vi "Log.vi"(8 "error in (no error)":errorcluster, 10 "Log Text":string, 11 "TDMS in":refnum<class "TDMS Sink.lvclass">) -> (0 "error out":errorcluster, 3 "TDMS out":refnum<class "TDMS Sink.lvclass">)   [LabVIEW 2020, in "LV Log.lvlib" / "TDMS Sink.lvclass"]
uses:
  TDMS Sink.lvclass
  TDMS Sink.lvclass/TDMS Sink.ctl
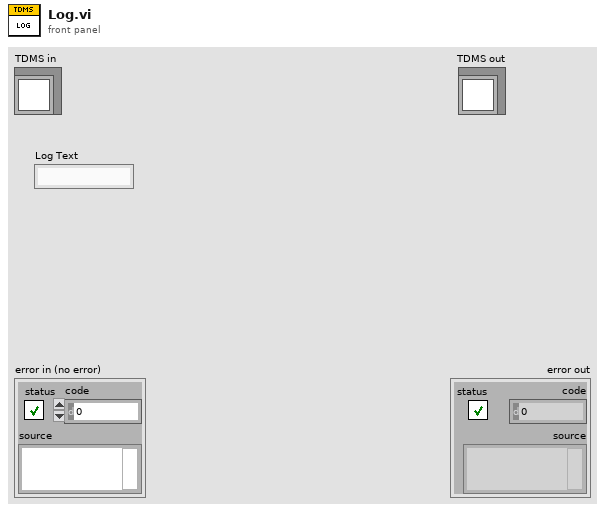
[diagram p1: front panel]
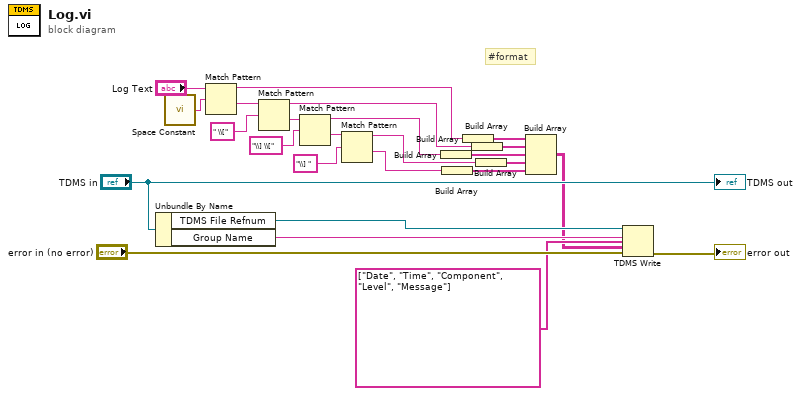
[diagram p0: block diagram]
diagram:
  # "#format"
  n1 = Unbundle By Name("TDMS in") -> ("TDMS File Refnum"=w22:refnum<k34>, "Group Name"=w21:string)
  n2 = call <vilib>:"Space Constant.vi"() -> ("String"=w12:string)
  n3 = Match Pattern(string="Log Text", regular expression=w12) -> (before substring=w13:string, after substring=w11:string)  [unwired: 1 in, 2 out]
  n4 = Match Pattern(string=w11, regular expression=" \\[") -> (before substring=w10:string, after substring=w8:string)  [unwired: 1 in, 2 out]
  n5 = Match Pattern(string=w8, regular expression="\\] \\[") -> (before substring=w6:string, after substring=w5:string)  [unwired: 1 in, 2 out]
  n6 = Match Pattern(string=w5, regular expression="\\] ") -> (before substring=w3:string, after substring=w2:string)  [unwired: 1 in, 2 out]
  n7 = Build Array(w6) -> (w16:string[])
  n8 = Build Array(w2) -> (w14:string[])
  n9 = Build Array(w13) -> (w18:string[])
  n10 = Build Array(w10) -> (w17:string[])
  n11 = Build Array(w3) -> (w15:string[])
  n12 = Build Array(w18, w17, w16, w15, w14) -> (w19:string[][])
  n13 = TDMS Write(0:w22, 5:w21, 7:string[] ["Date", "Time", "Component", "Level", "Message"] ("channel name(s) in (Untitled)"), 9:w19, 11:"error in (no error)") -> (15:→"error out":errorcluster)  [unwired: 1 in, 3 out]
  "TDMS out" <- "TDMS in"
